vi "Process Data2D.vi"(8 "error in (no error)":errorcluster, 10 "Data2D in":refnum<class "Data2D.lvclass">, 11 "ThresholdProcess2D in":refnum<class "ThresholdProcessor2D.lvclass">) -> (0 "error out":errorcluster, 2 "Data2D out":refnum<class "Data2D.lvclass">, 3 "ThresholdProcess2D out":refnum<class "ThresholdProcessor2D.lvclass">)   [LabVIEW 2014, in "ThresholdProcessor2D.lvclass"]
uses:
  ThresholdProcessor2D.lvclass
  Framework/Model/Data/Data2D/Data2D.lvclass
  ThresholdProcessor2D.lvclass/ThresholdProcessor2D.ctl
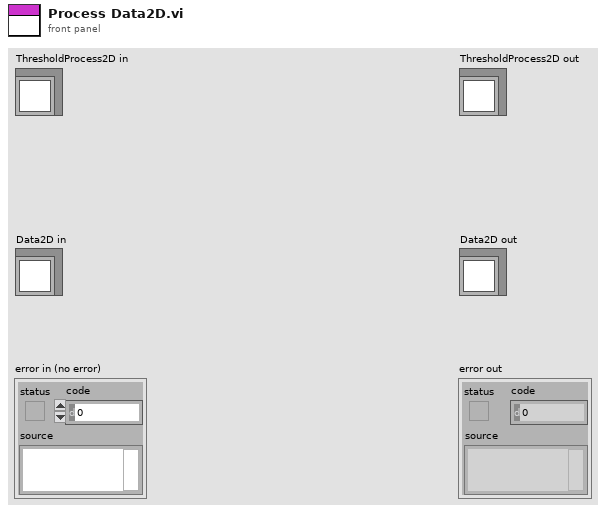
[diagram p1: front panel]
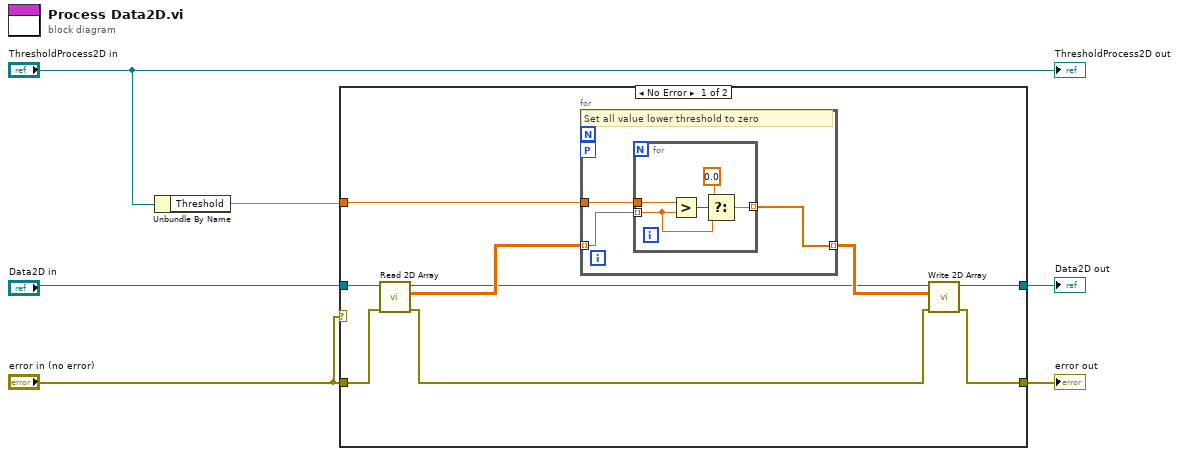
[diagram p0: block diagram]
diagram:
  n1 = Unbundle By Name("ThresholdProcess2D in") -> ("Threshold"=w3:dbl)
  n2 = case shown="No Error" "error in (no error)" {
    tunnel: "error in (no error)" -> [w15 w25]
    tunnel: [w13 w25] -> w6
    tunnel: [w12 w24] -> w1
    tunnel: "Data2D in" -> [w11 w24]
    tunnel: w3 -> [w8 _]
    frame No Error {
      n3 = call "Read 2D Array.vi"("error in (no error)"=w15, "Data2D in"=w11) -> ("error out"=w14:errorcluster, "2D Array"=w10:dbl[][], "Data2D out"=w7:refnum<class "Data2D.lvclass">)  [unwired: 7 in]
      n4 = for {
        tunnel: w10 -> [w16] mode=indexing
        tunnel: [w17] -> w9 mode=indexing
        tunnel: w8 -> [w18]
        workers-P: _ -> [_]
        # "Set all value lower threshold to zero"
        n5 = for {
          tunnel: w18 -> [w22]
          tunnel: [w21] -> w17 mode=indexing
          tunnel: w16 -> [w20] mode=indexing
          n6 = Greater?(x=w22, y=w20) -> (0:w23:bool)
          n7 = Select(t=0.0, s=w23, f=w20) -> (s? t:f=w21:dbl)
        }
      }
      n8 = call "Write 2D Array.vi"("error in (no error)"=w14, "2D Array"=w9, "Data2D in"=w7) -> ("error out"=w13:errorcluster, "Data2D out"=w12:refnum<class "Data2D.lvclass">)  [unwired: 7 in]
    }
    frame Error {
    }
  }
  "error out" <- w6
  "Data2D out" <- w1
  "ThresholdProcess2D out" <- "ThresholdProcess2D in"
